vi "Advanced Sequence and RefTrigger.vi"() -> ()   [LabVIEW 2023]
uses:
  <instrlib>/niDCPower/nidcpower.llb/niDCPower Sequence Attribute Type.ctl
  <instrlib>/niDCPower/nidcpower.llb/niDCPower Output Function.ctl
  <instrlib>/niDCPower/nidcpower.llb/niDCPower Source Mode.ctl
  <instrlib>/niDCPower/nidcpower.llb/niDCPower Wait For Event - Event.ctl
  <instrlib>/niDCPower/nidcpower.llb/niDCPower Export Signal - Signal.ctl
  <instrlib>/niDCPower/nidcpower.llb/niDCPower Send Software Edge Trigger - Signal.ctl
  <instrlib>/niScope/Controls/niScope trigger source digital.ctl
  <instrlib>/niScope/Controls/niScope trigger slope.ctl
  <instrlib>/niDCPower/nidcpower.llb/niDCPower Get Channel Name From String.vi
  <instrlib>/niDCPower/nidcpower.llb/niDCPower Create Advanced Sequence Step With Channels.vi
  <instrlib>/niScope/Utility/niScope Get Channel Name From String.vi
  <instrlib>/niScope/Configure/Trigger/niScope Configure Trigger Digital.vi
  <instrlib>/niScope/Acquire/Fetch/niScope Multi Fetch Cluster.vi
  <instrlib>/niScope/Configure/Trigger/niScope Configure Trigger Window.vi
  <instrlib>/niScope/Configure/Trigger/niScope Configure Trigger Edge.vi
panel:
  out "error out":errorcluster
  out "voltage measurements":dbl[](array[numeric]) caption="SMU measurements"
  in  "HW Sequence Steps":T1(array[cluster])=[{"Voltage Level"=0.1, "Aperture Time Array (Sec)"=0.016}, {"Voltage Level"=1.0, "Aperture Time Array (Sec)"=0.016}, {"Voltage Level"=2.0, "Aperture Time Array (Sec)"=0.016}] {"Aperture Time Array (Sec)" format="%#_6p"}
  in  "Source Delay (Sec)":dbl=0.1 format="%.3p"
  in  "SMU Name":refnum<k15>="SMU_4162_C02_S02" caption="SMU Resource Name"
  out "Waveform(s)":T2(graph)
  in  "Reference Position":dbl=50.0 caption="Ref Position" format="%#.1f"
  in  "Scope Name":refnum<k15>="Scope_5152_C02_S05" caption="Scope  Name(s)"
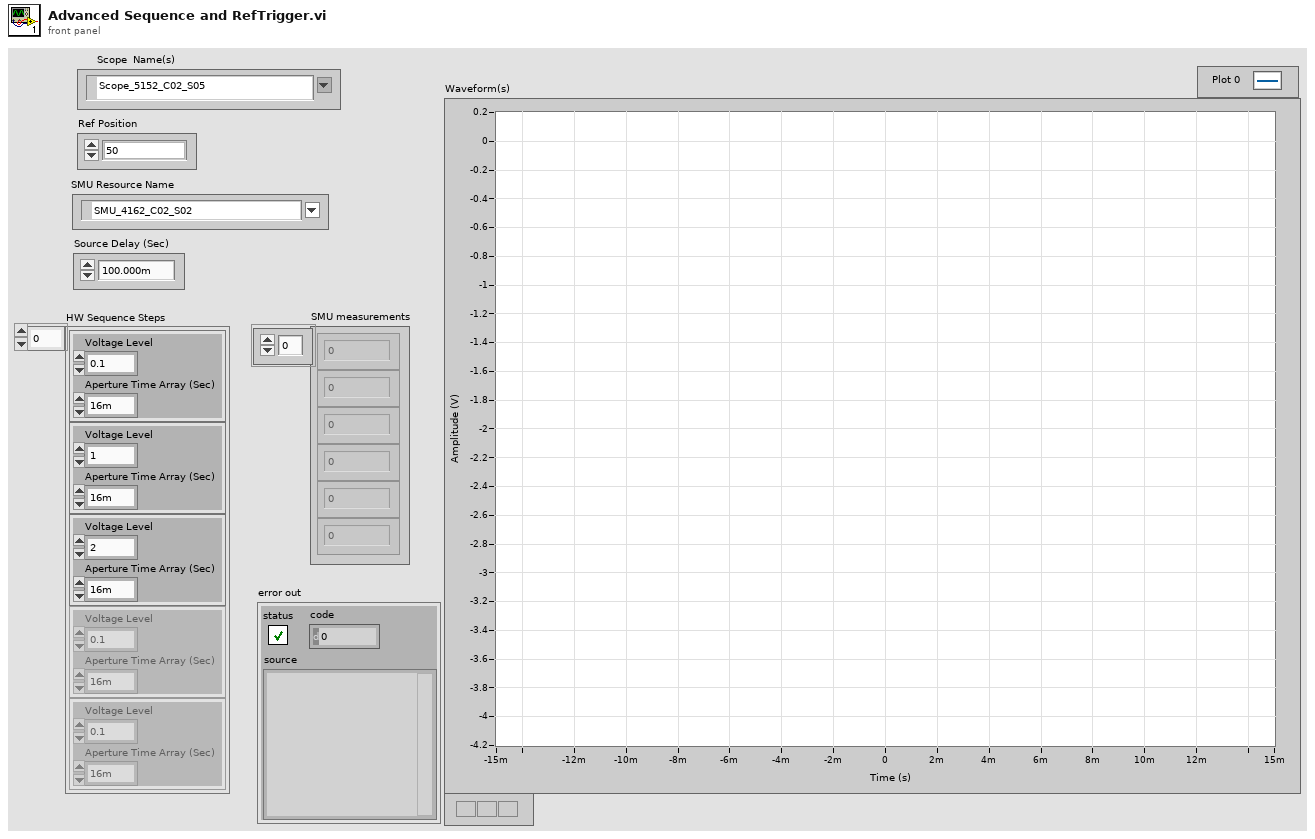
[diagram p1: front panel]
types:
  T1 = cluster{"Voltage Level":dbl, "Aperture Time Array (Sec)":dbl}[]
  T2 = cluster{"relativeInitialX":dbl, "xIncrement":dbl, "wfm":dbl[]}[]
  T3 = typedef "niDCPower Export Signal - Signal.ctl" = i32
  T4 = typedef "niDCPower Send Software Edge Trigger - Signal.ctl" = i32
  T5 = typedef "niDCPower Wait For Event - Event.ctl" = i32
  T6 = typedef "niDCPower Source Mode.ctl" = i32
  T7 = typedef "niDCPower Output Function.ctl" = i32
  T8 = typedef "niDCPower Sequence Attribute Type.ctl" = i32
  T9 = typedef "niScope trigger source digital.ctl" = string
  T10 = typedef "niScope trigger slope.ctl" = i32
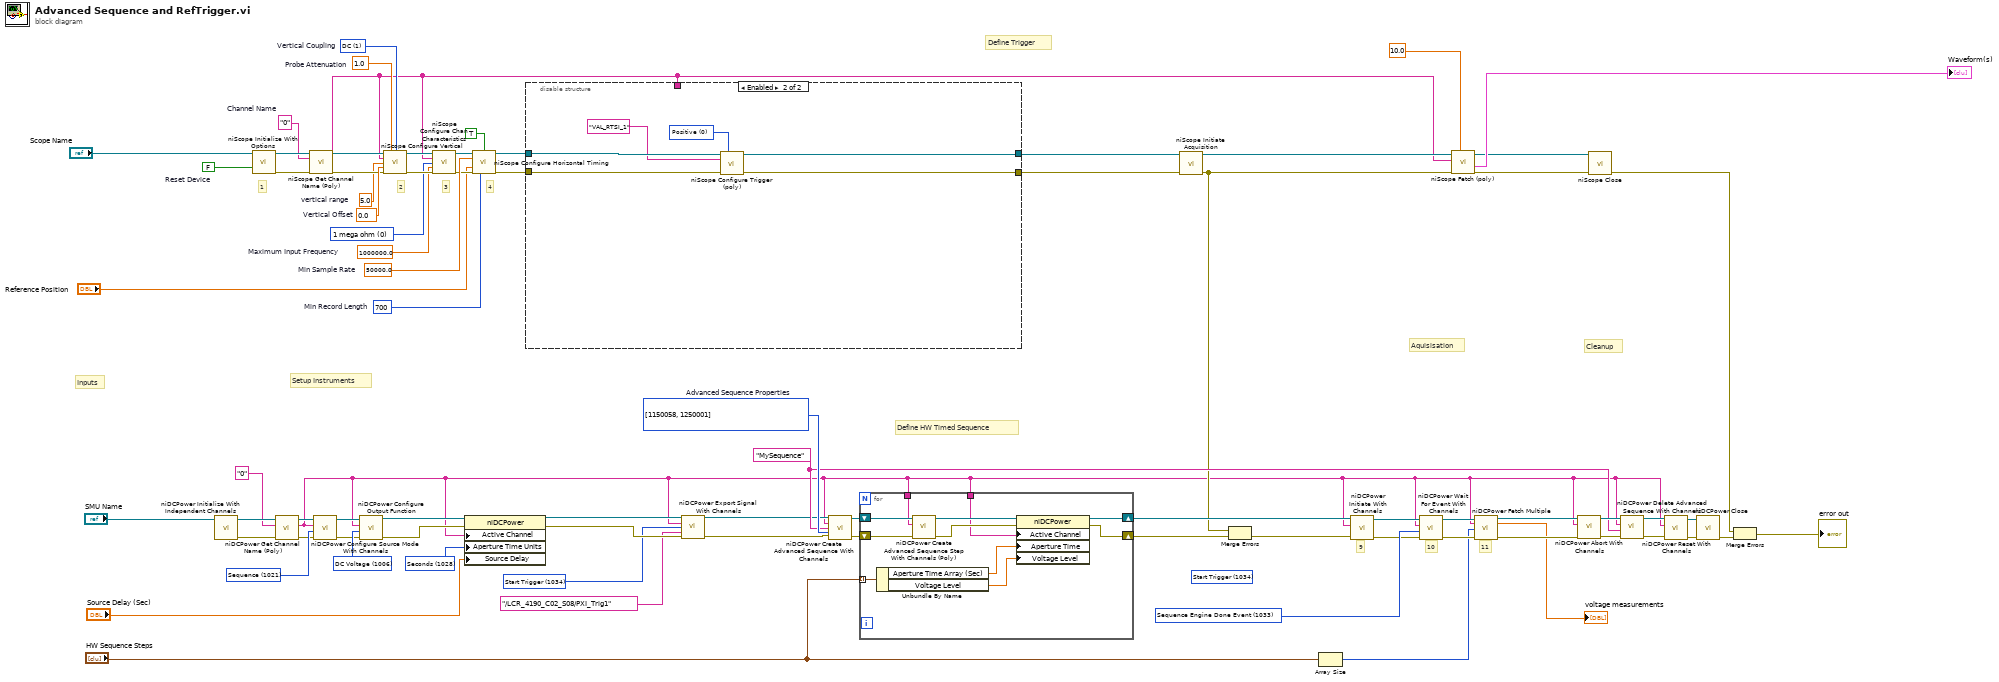
[diagram p0: block diagram]
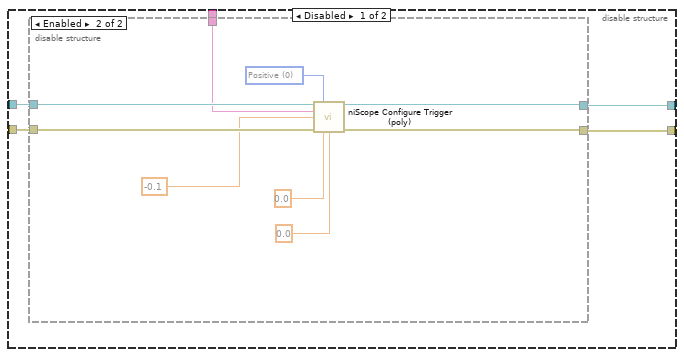
[diagram p2: hidden frame]
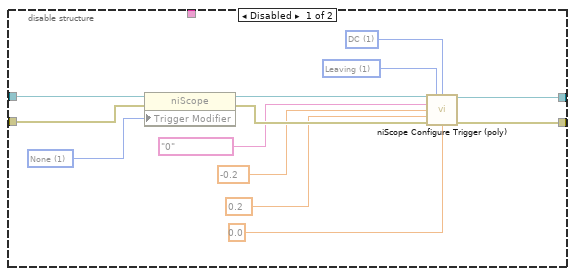
[diagram p3: hidden frame]
diagram:
  w3 = T3 1034 items=["Source Complete Event"=1030, "Measure Complete Event"=1031, "Sequence Iteration Complete Event"=1032, "Sequence Engine Done Event"=1033, "Pulse Complete Event"=1051, "Ready For Pulse Trigger Event"=1052, "Start Trigger"=1034, "Source Trigger"=1035, "Measure Trigger"=1036, "Sequence Advance Trigger"=1037, "Pulse Trigger"=1053] ("signal")
  w27 = "0"  # Channel Name
  (unwired) T4 1034 items=["Start Trigger"=1034, "Source Trigger"=1035, "Measure Trigger"=1036, "Sequence Advance Trigger"=1037, "Pulse Trigger"=1053, "Shutdown Trigger"=1118] ("signal")
  w39 = 1.0  # Probe Attenuation
  w45 = 700  # Min Record Length
  w46 = 50000.0  # Min Sample Rate
  w38 = 1000000.0  # Maximum Input Frequency
  w33 = 1 items=["AC", "DC", "Ground"]  # Vertical Coupling
  w40 = 0.0  # Vertical Offset
  w25 = 5.0  # vertical range
  w26 = u32 0 items=["1 mega ohm"=0, "50 ohms"=2] ("input impedance")
  w65 = 1028 items=["Seconds"=1028, "Power Line Cycles"=1029] ("Measurement:Aperture Time Units")
  w48 = "MySequence" ("sequence name")
  w67 = T5 1033 items=["Source Complete Event"=1030, "Measure Complete Event"=1031, "Sequence Iteration Complete Event"=1032, "Sequence Engine Done Event"=1033] ("event")
  w71 = T6 1021 items=["Single Point"=1020, "Sequence"=1021] ("source mode")
  w62 = T7 1006 items=["DC Voltage"=1006, "DC Current"=1007] ("output function")
  w52 = T8[] [1150058, 1250001] items=["Source -> Output Function"=1150008, "Source -> Output Enabled"=1250006, "Source -> Output Resistance"=1150061, "Source -> Transient Response"=1150062, "Source -> Custom Transient Response -> Voltage Gain Bandwidth"=1150067, "Source -> Custom Transient Response -> Voltage Compensation Frequency"=1150068, "Source -> Custom Transient Response -> Voltage Pole-Zero Ratio"=1150069, "Source -> Custom Transient Response -> Current Gain Bandwidth"=1150070, "Source -> Custom Transient Response -> Current Compensation Frequency"=1150071, "Source -> Custom Transient Response -> Current Pole-Zero Ratio"=1150072, "Source -> DC Voltage -> Voltage Level"=1250001, "Source -> DC Voltage -> Voltage Level Range"=1150005, "Source -> DC Voltage -> Current Limit"=1250005, "Source -> DC Voltage -> Current Limit High"=1150187, "Source -> DC Voltage -> Current Limit Low"=1150188, "Source -> DC Voltage -> Current Limit Range"=1150004, "Source -> DC Current -> Current Level"=1150009, "Source -> DC Current -> Current Level Range"=1150011, "Source -> DC Current -> Voltage Limit"=1150010, "Source -> DC Current -> Voltage Limit High"=1150185, "Source -> DC Current -> Voltage Limit Low"=1150186, "Source -> DC Current -> Voltage Limit Range"=1150012, "Source -> DC Current -> Current Level Slew Rate -> Rising"=1150343, "Source -> DC Current -> Current Level Slew Rate -> Falling"=1150344, "Source -> Pulse Voltage -> Pulse Voltage Level"=1150080, "Source -> Pulse Voltage -> Pulse Bias Voltage Level"=1150082, "Source -> Pulse Voltage -> Pulse Voltage Level Range"=1150084, "Source -> Pulse Voltage -> Pulse Current Limit"=1150081, "Source -> Pulse Voltage -> Pulse Current Limit High"=1150193, "Source -> Pulse Voltage -> Pulse Current Limit Low"=1150194, "Source -> Pulse Voltage -> Pulse Bias Current Limit"=1150083, "Source -> Pulse Voltage -> Pulse Bias Current Limit High"=1150195, "Source -> Pulse Voltage -> Pulse Bias Current Limit Low"=1150196, "Source -> Pulse Voltage -> Pulse Current Limit Range"=1150085, "Source -> Pulse Current -> Pulse Current Level"=1150086, "Source -> Pulse Current -> Pulse Bias Current Level"=1150088, "Source -> Pulse Current -> Pulse Current Level Range"=1150090, "Source -> Pulse Current -> Pulse Voltage Limit"=1150087, "Source -> Pulse Current -> Pulse Voltage Limit High"=1150189, "Source -> Pulse Current -> Pulse Voltage Limit Low"=1150190, "Source -> Pulse Current -> Pulse Bias Voltage Limit"=1150089, "Source -> Pulse Current -> Pulse Bias Voltage Limit High"=1150191, "Source -> Pulse Current -> Pulse Bias Voltage Limit Low"=1150192, "Source -> Pulse Current -> Pulse Voltage Limit Range"=1150091, "Source -> Advanced -> Source Delay"=1150051, "Source -> Advanced -> Pulse Bias Delay"=1150092, "Source -> Advanced -> Pulse On Time"=1150093, "Source -> Advanced -> Pulse Off Time"=1150094, "Source -> Advanced -> OVP Enabled"=1250002, "Source -> Advanced -> OVP Limit"=1250003, "Source -> Advanced -> Compliance Limit Symmetry"=1150184, "Source -> Advanced -> Sequence Step Delta Time"=1150198, "Source -> Advanced -> Conduction Voltage -> Mode"=1150350, "Source -> Advanced -> Conduction Voltage -> On Threshold"=1150351, "Source -> Advanced -> Conduction Voltage -> Off Threshold"=1150352, "Measurement -> Sense"=1150013, "Measurement -> Aperture Time"=1150058, "Measurement -> Measure Record Length"=1150063, "Measurement -> Advanced -> DC Noise Rejection"=1150066, "Measurement -> Autorange"=1150244, "Measurement -> Advanced -> Autorange Behavior"=1150245, "Measurement -> Advanced -> Autorange Aperture Time Mode"=1150246, "Measurement -> Advanced -> Autorange Minimum Aperture Time"=1150247, "Measurement -> Advanced -> Autorange Minimum Aperture Time Units"=1150248, "Measurement -> Advanced -> Autorange Minimum Current Range"=1150255, "Measurement -> Advanced -> Autorange Minimum Voltage Range"=1150256, "Measurement -> Advanced -> Autorange Threshold Mode"=1150257, "Measurement -> Advanced -> Autorange Maximum Delay After Range Change"=1150322, "LCR -> Instrument Mode"=1150208, "LCR -> Source Delay Mode"=1150315, "LCR -> Measurement Time"=1150218, "LCR -> Custom Measurement Time"=1150258, "LCR -> AC Stimulus -> Function"=1150209, "LCR -> AC Stimulus -> Frequency"=1150210, "LCR -> AC Stimulus -> Voltage Amplitude"=1150211, "LCR -> AC Stimulus -> Current Amplitude"=1150212, "LCR -> AC Stimulus -> Advanced -> Voltage Range"=1150265, "LCR -> AC Stimulus -> Advanced -> Current Range"=1150267, "LCR -> AC Stimulus -> Advanced -> Source Aperture Time"=1150349, "LCR -> DC Bias -> Source"=1150213, "LCR -> DC Bias -> Voltage Level"=1150214, "LCR -> DC Bias -> Current Level"=1150215, "LCR -> DC Bias -> Advanced -> Voltage Range"=1150266, "LCR -> DC Bias -> Advanced -> Current Range"=1150274, "LCR -> DC Bias -> Advanced -> Transient Response"=1150347, "LCR -> Compensation -> Open -> Enabled"=1150220, "LCR -> Compensation -> Open -> Conductance"=1150261, "LCR -> Compensation -> Open -> Susceptance"=1150262, "LCR -> Compensation -> Short -> Enabled"=1150221, "LCR -> Compensation -> Short -> Resistance"=1150263, "LCR -> Compensation -> Short -> Reactance"=1150264, "LCR -> Compensation -> Load -> Enabled"=1150222, "LCR -> Compensation -> Load -> Measured Resistance"=1150268, "LCR -> Compensation -> Load -> Measured Reactance"=1150269, "LCR -> Compensation -> Load -> Actual Resistance"=1150270, "LCR -> Compensation -> Load -> Actual Reactance"=1150271, "LCR -> Impedance Range -> Impedance Range"=1150217, "LCR -> Impedance Range -> Impedance Autorange"=1150216, "LCR -> Impedance Range -> Advanced -> Impedance Range Source"=1150321, "LCR -> Impedance Range -> Advanced -> Load Resistance"=1150318, "LCR -> Impedance Range -> Advanced -> Load Inductance"=1150319, "LCR -> Impedance Range -> Advanced -> Load Capacitance"=1150320]  # Advanced Sequence Properties
  w79 = FALSE  # Reset Device
  # "Inputs"
  # "Setup Instruments"
  # "Define HW Timed Sequence"
  # "Define Trigger"
  # "Aquisisation"
  # "Cleanup"
  # "2"
  # "3"
  # "4"
  # "9"
  # "11"
  # "10"
  # "1"
  n1 = call <instrlib>:"niDCPower Initialize With Independent Channels.vi"("resource name"="SMU Name") -> ("error out"=w50:errorcluster, "instrument handle out"=w72:refnum<k15>)  [unwired: 9 in]
  n2 = call <instrlib>:"niScope Initialize With Options.vi"("resource name"="Scope Name", "reset device"=w79) -> ("instrument handle"=w78:refnum<k15>, "error out"=w76:errorcluster)  [unwired: 12 in]
  n3 = call-poly <instrlib>:"niDCPower Get Channel Name (Poly).vi"("error in (no error)"=w50, "index"="0", "instrument handle"=w72) -> ("error out"=w49:errorcluster, "name"=w2:string, "instrument handle out"=w51:refnum<k15>)  [unwired: 6 in]
  n4 = call-poly <instrlib>:"niScope Get Channel Name (Poly).vi"("instrument handle"=w78, "index"=w27, "error in"=w76) -> ("instrument handle out"=w29:refnum<k15>, "channel name"=w9:string, "error out"=w28:errorcluster)  [unwired: 10 in]
  n5 = call <instrlib>:"niDCPower Configure Source Mode With Channels.vi"("error in (no error)"=w49, "source mode"=w71, "channel name"=w2, "instrument handle"=w51) -> ("error out"=w54:errorcluster, "instrument handle out"=w53:refnum<k15>)  [unwired: 6 in]
  n6 = call <instrlib>:"niDCPower Configure Output Function.vi"("error in (no error)"=w54, "output function"=w62, "channel name"=w2, "instrument handle"=w53) -> ("error out"=w19:errorcluster, "instrument handle out"=w18:refnum<k15>)  [unwired: 6 out]
  n7 = call <instrlib>:"niScope Configure Vertical.vi"("instrument handle"=w29, "probe attenuation"=w39, "vertical coupling"=w33, "channels"=w9, "vertical range"=w25, "vertical offset"=w40, "error in"=w28) -> ("instrument handle out"=w44:refnum<k15>, "error out"=w43:errorcluster)  [unwired: 7 in]
  n8 = call <instrlib>:"niScope Configure Chan Characteristics.vi"("instrument handle"=w44, "channels"=w9, "input impedance"=w26, "maximum input frequency"=w38, "error in"=w43) -> ("instrument handle out"=w41:refnum<k15>, "error out"=w42:errorcluster)  [unwired: 9 in]
  n9 = property class="niDCPower"(reference=w18, error in=w19, "Active Channel"=w2, "Aperture Time Units"=w65, "Source Delay"="Source Delay (Sec)") -> (reference out=w5:refnum<k15>, error out=w8:errorcluster)
  n10 = call <instrlib>:"niScope Configure Horizontal Timing.vi"("instrument handle"=w41, "enforce realtime"=TRUE ("Enforce Realtime"), "min sample rate"=w46, "reference position"="Reference Position", "error in"=w42, "min record length"=w45) -> ("instrument handle out"=w32:refnum<k15>, "error out"=w31:errorcluster)  [unwired: 8 in]
  n11 = disable-structure shown="Enabled" {
    disable-tunnel: [w84 w111] -> w35
    disable-tunnel: [w83 w110] -> w34
    disable-tunnel: w32 -> [w82 w112]
    disable-tunnel: w31 -> [w81 w109]
    disable-tunnel: w9 -> [w80 _]
    frame Disabled {
      n12 = disable-structure shown="Enabled" {
        disable-tunnel: [w96 w104] -> w84
        disable-tunnel: [w95 w100] -> w83
        disable-tunnel: w82 -> [w94 w106]
        disable-tunnel: w81 -> [w93 w105]
        disable-tunnel: w80 -> [_ w99]
        frame Disabled {
          w88 = 1 items=["Entering", "Leaving"] ("Window Mode")
          w86 = u16 1 items=["AC"=0, "DC"=1, "HF Reject"=3, "LF Reject"=4, "AC Plus HF Reject"=1001] ("Coupling 2")
          w90 = 1 items=["None"=1, "Auto Trigger"=2] ("Triggering:Trigger Modifier")
          n13 = property on="Property Node" class="niScope"(reference=w94, error in=w93, "Trigger Modifier"=w90) -> (reference out=w91:refnum<k15>, error out=w92:errorcluster)
          n14 = call-poly <instrlib>:"niScope Configure Trigger (poly).vi"("instrument handle"=w91, "trigger window mode"=w88, "trigger coupling"=w86, "trigger source"="0" ("Trigger Source 3"), "low level"=-0.2 ("Low Level"), "high level"=0.2 ("High Level"), "error in"=w92, "trigger delay"=0.0 ("Trigger Delay")) -> ("instrument handle out"=w96:refnum<k15>, "error out"=w95:errorcluster)  [unwired: 6 in]
        }
        frame Enabled {
          w103 = T10 0 items=["Positive", "Negative"] ("trigger slope")
          n15 = call-poly <instrlib>:"niScope Configure Trigger (poly).vi"("instrument handle"=w106, "trigger slope"=w103, "trigger source"=w99, "trigger level"=-0.1, "error in"=w105, "trigger holdoff"=0.0, "trigger delay"=0.0) -> ("instrument handle out"=w104:refnum<k15>, "error out"=w100:errorcluster)  [unwired: 7 in]
        }
      }
    }
    frame Enabled {
      w107 = T10 0 items=["Positive", "Negative"] ("trigger slope")
      n16 = call-poly <instrlib>:"niScope Configure Trigger (poly).vi"("instrument handle"=w112, "trigger slope"=w107, "trigger source"=T9 "VAL_RTSI_1", "error in"=w109) -> ("instrument handle out"=w111:refnum<k15>, "error out"=w110:errorcluster)  [unwired: 10 in]
    }
  }
  n17 = call <instrlib>:"niDCPower Export Signal With Channels.vi"("instrument handle"=w5, "channel name"=w2, "signal"=w3, "output terminal"=tag "/LCR_4190_C02_S08/PXI_Trig1", "error in (no error)"=w8) -> ("instrument handle out"=w6:refnum<k15>, "error out"=w7:errorcluster)  [unwired: 9 in]
  n18 = call <instrlib>:"niDCPower Create Advanced Sequence With Channels.vi"("instrument handle"=w6, "channel name"=w2, "sequence name"=w48, "advanced sequence properties"=w52, "error in (no error)"=w7) -> ("instrument handle out"=w64:refnum<k15>, "error out"=w63:errorcluster)  [unwired: 9 in]
  n19 = for {
    shift-right: [w120] -> w20
    shift-left: w63 -> [w123]
    shift-right: [w119] -> w14
    shift-left: w64 -> [w118]
    tunnel: "HW Sequence Steps" -> [w115] mode=indexing
    tunnel: w2 -> [w117]
    tunnel: w2 -> [w116]
    n20 = Unbundle By Name(w115) -> ("Aperture Time Array (Sec)"=w114:dbl, "Voltage Level"=w113:dbl)
    n21 = call-poly <instrlib>:"niDCPower Create Advanced Sequence Step With Channels (Poly).vi"("error in (no error)"=w123, "channel name"=w117, "instrument handle"=w118) -> ("error out"=w121:errorcluster, "instrument handle out"=w122:refnum<k15>)  [unwired: 7 in]
    n22 = property class="niDCPower"(reference=w122, error in=w121, "Active Channel"=w116, "Aperture Time"=w114, "Voltage Level"=w113) -> (reference out=w119:refnum<k15>, error out=w120:errorcluster)
  }
  n23 = call <instrlib>:"niScope Initiate Acquisition.vi"("instrument handle"=w35, "error in"=w34) -> ("instrument handle out"=w10:refnum<k15>, "error out"=w11:errorcluster)  [unwired: 12 in]
  n24 = Merge Errors(w11, w20) -> (w15:errorcluster)
  n25 = Array Size(array="HW Sequence Steps") -> (size(s)=w55:i32)
  n26 = call <instrlib>:"niDCPower Initiate With Channels.vi"("error in (no error)"=w15, "channel name"=w2, "instrument handle"=w14) -> ("error out"=w13:errorcluster, "instrument handle out"=w70:refnum<k15>)  [unwired: 7 in]
  n27 = call <instrlib>:"niDCPower Wait For Event With Channels.vi"("error in (no error)"=w13, "event"=w67, "channel name"=w2, "instrument handle"=w70) -> ("error out"=w68:errorcluster, "instrument handle out"=w69:refnum<k15>)  [unwired: 6 in]
  n28 = call-poly <instrlib>:"niScope Fetch (poly).vi"("timeout"=10.0, "error in"=w11, "channels"=w9, "instrument handle"=w10) -> ("error out"=w21:errorcluster, "waveform"=→"Waveform(s)":T2, "instrument handle out"=w22:refnum<k15>)  [unwired: 4 in, 1 out]
  n29 = call <instrlib>:"niDCPower Fetch Multiple.vi"("instrument handle"=w69, "channel name"=w2, "count (1)"=w55, "error in (no error)"=w68) -> ("instrument handle out"=w61:refnum<k15>, "voltage measurements"=→"voltage measurements":dbl[], "error out"=w60:errorcluster)  [unwired: 6 in, 3 out]
  n30 = call <instrlib>:"niDCPower Abort With Channels.vi"("error in (no error)"=w60, "channel name"=w2, "instrument handle"=w61) -> ("error out"=w58:errorcluster, "instrument handle out"=w59:refnum<k15>)  [unwired: 7 in]
  n31 = call <instrlib>:"niScope Close.vi"("instrument handle"=w22, "error in"=w21) -> ("error out"=w23:errorcluster)  [unwired: 13 in]
  n32 = call <instrlib>:"niDCPower Delete Advanced Sequence With Channels.vi"("error in (no error)"=w58, "sequence name"=w48, "channel name"=w2, "instrument handle"=w59) -> ("error out"=w56:errorcluster, "instrument handle out"=w57:refnum<k15>)  [unwired: 6 in]
  n33 = call <instrlib>:"niDCPower Reset With Channels.vi"("error in (no error)"=w56, "channel name"=w2, "instrument handle"=w57) -> ("error out"=w73:errorcluster, "instrument handle out"=w74:refnum<k15>)  [unwired: 7 in]
  n34 = call <instrlib>:"niDCPower Close.vi"("error in (no error)"=w73, "instrument handle"=w74) -> ("error out"=w24:errorcluster)  [unwired: 9 out]
  n35 = Merge Errors(w23, w24) -> (→"error out":errorcluster)
